vi "Fix file path.vi"(4 "input path":string, 5 "replacement (-)":string=" ") -> (0 "error out":errorcluster, 1 "corrected path":string)   [LabVIEW 2021, in "MatS Libs.lvlib"]
doc: "Wrapper to Search and replace string.vi that replaces invalid characters in file path/name with valid a character.\nParams:\nReplacement - default is \"space\""
uses:
  <userlib>/MatS Libs/MatS Libs.lvlib
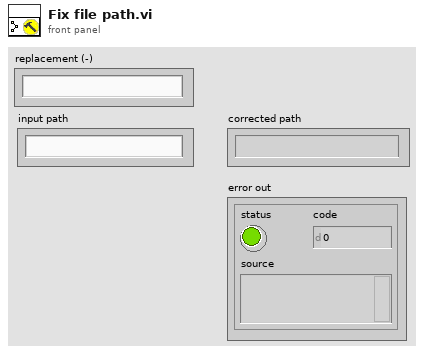
[diagram p1: front panel]
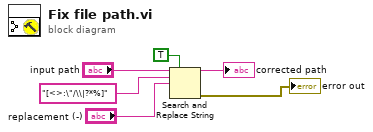
[diagram p0: block diagram]
diagram:
  n1 = Search and Replace String(replace all?=TRUE ("replace all? (F)"), input string="input path", search string="[<>:\"/\\|?*%]" ("regular expression"), replace string="replacement (-)") -> (result string=→"corrected path":string, error out=→"error out":errorcluster)  [unwired: 4 in, 2 out]
